vi "Server_REPL_Script.vi"(8 "error in (no error)":errorcluster, 9 "Code":string, 11 "Server":path) -> (0 "error out":errorcluster)   [LabVIEW 2020]
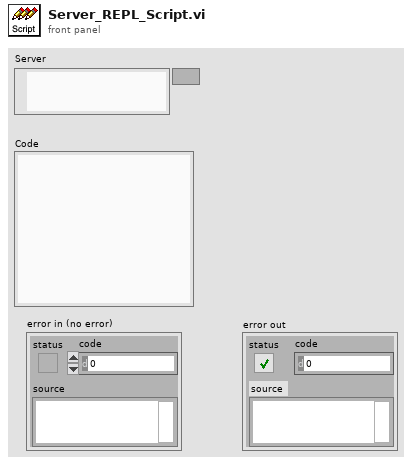
[diagram p1: front panel]
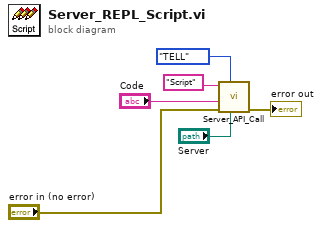
[diagram p0: block diagram]
diagram:
  n1 = call "Server_API_Call.vi"("Server"="Server", "Direction"=enum16{"ASK", "TELL"}."TELL", "error in (no error)"="error in (no error)", "Payload"="Code", "cmd"="Script" ("url")) -> ("error out"=→"error out":errorcluster)  [unwired: 3 in, 3 out]
